vi "To String (Array).vi"(6 "pretty print? (T)":bool=TRUE, 7 "enable LabVIEW extensions? (T)":bool=TRUE, 8 "error in (no error)":errorcluster, 11 "JSON Value in":refnum<class "JSON Value.lvclass">) -> (0 "error out":errorcluster, 3 "String":string)   [LabVIEW 2016, in "JSON Value.lvclass"]
doc: "Flattens the given JSON data to a string."
uses:
  JSON Value.lvclass
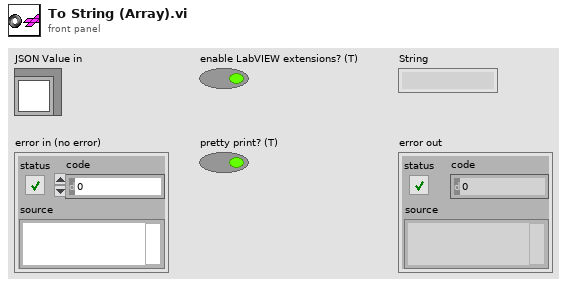
[diagram p1: front panel]
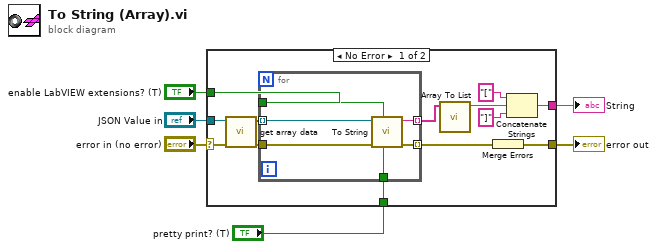
[diagram p0: block diagram]
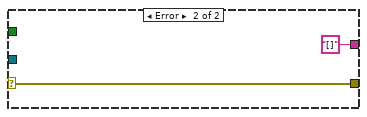
[diagram p2: hidden frame]
diagram:
  n1 = case shown="No Error" "error in (no error)" {
    selector: "error in (no error)" -> [w9 w27]
    tunnel: "JSON Value in" -> [w11 _]
    tunnel: [w17 w27] -> w4
    tunnel: [w16 "[]"] -> w3
    tunnel: "enable LabVIEW extensions? (T)" -> [w12 _]
    tunnel: "pretty print? (T)" -> [w7 _]
    frame No Error {
      n2 = call "get array data.vi"("error in (no error)"=w9, "JSON Value in"=w11) -> ("error out"=w8:errorcluster, "JSON Array out"=w10:refnum<class "JSON Value.lvclass">[])  [unwired: 8 in]
      n3 = for {
        tunnel: [w25] -> w19 mode=indexing
        tunnel: w8 -> [w24]
        tunnel: [w23] -> w18 mode=indexing
        tunnel: w12 -> [w22]
        tunnel: w10 -> [w21] mode=indexing
        tunnel: w7 -> [w20]
        n4 = call "To String.vi"("pretty print? (T)"=w20, "enable LabVIEW extensions? (T)"=w22, "error in (no error)"=w24, "JSON Value in"=w21) -> ("error out"=w23:errorcluster, "String"=w25:string)  [unwired: 6 in]
      }
      n5 = call "Array To List.vi"("Array"=w19) -> ("String"=w15:string)  [unwired: 10 in]
      n6 = Merge Errors(w18) -> (w17:errorcluster)
      n7 = Concatenate Strings("[" ("string"), w15, "]" ("string")) -> (w16:string)
    }
    frame Error {
    }
  }
  "String" <- w3
  "error out" <- w4
